vi "Test 100000 Log Writes.vi"(11 "Test Case In":refnum<class "File Sink.lvclass">) -> (0 "error out":errorcluster, 3 "Test Case Out":refnum<class "File Sink.lvclass">)   [LabVIEW 2020, in "Testing.lvlib" / "File Sink.lvclass"]
uses:
  File Sink.lvclass
  C:/Program Files (x86)/National Instruments/LabVIEW 2020/vi.lib/Astemes/LUnit/Test Case.lvclass
  Source/Type Defs/Debug Level.ctl
  <vilib>/Astemes/LUnit/Test Case.lvclass/Test Case.ctl
  0e3525c7-7213-410e-b7d5-902f6b8fb3e7.vi
  7c7b706d-9091-48de-aeff-4f50f38094d5.vi
  <vilib>/Astemes/LUnit/Core/LUnit Test Case/Private/Append Pass Result.vi
  <vilib>/Astemes/LUnit/Core/LUnit Test Case/Private/Append Fail Result.vi
  0e3525c7-7213-410e-b7d5-902f6b8fb3e7.vi/9c5d11cd-9439-4240-a1ee-d9baace9c924.vi
  7c7b706d-9091-48de-aeff-4f50f38094d5.vi/9c5d11cd-9439-4240-a1ee-d9baace9c924.vi
  <vilib>/Astemes/LUnit/Core/LUnit Test Case/Private/Run In UI.vi
  <vilib>/Utility/error.llb/Clear Errors.vi
  Source/Sinks/File Sink/File Sink.lvclass
  C:/Users/hughe_cx/Documents/05_repos/LVLog/Source/Sinks/Sink/Sink.lvclass
  Source/LV Log.lvlib
  Source/Logger/Logger.lvclass
  Testing.lvlib
  <vilib>/Astemes/LUnit/Test Case.lvclass
panel:
  out "Iteration (of 100000)":i32
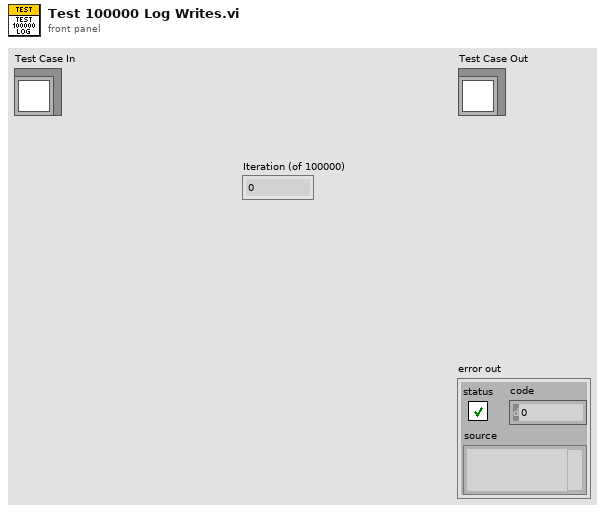
[diagram p1: front panel]
types:
  T1 = typedef "LV Log.lvlib/Debug Level.ctl" = enum16{"DEFAULT", "DEBUG", "INFO", "WARN", "ERROR", "FATAL"}
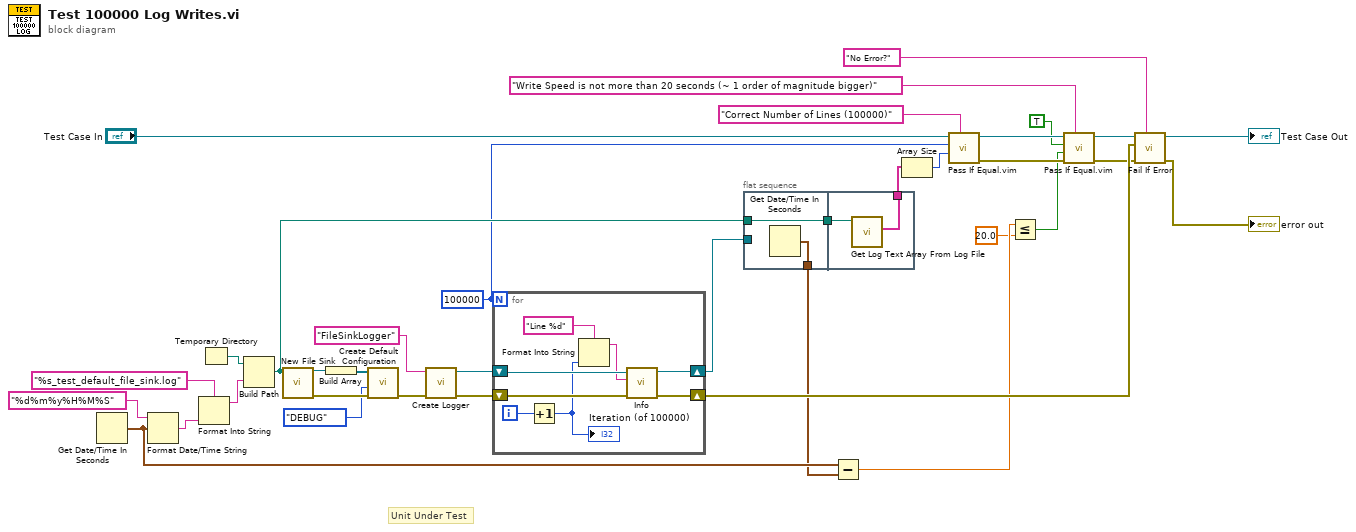
[diagram p0: block diagram]
diagram:
  w13 = 100000
  # "Unit Under Test"
  n1 = Get Date/Time In Seconds() -> (seconds since 1Jan1904=w7:timestamp)
  n2 = Format Date/Time String(time format string (%c)="%d%m%y%H%M%S", seconds (now)=w7) -> (date/time string=w28:string)  [unwired: 1 in]
  n3 = Format Into String(format string="%s_test_default_file_sink.log", w28) -> (resulting string=w30:string)  [unwired: 2 in, 1 out]
  n4 = Temporary Directory() -> (w32:path)
  n5 = Build Path(base path=w32, name or relative path=w30) -> (appended path=w23:path)
  n6 = call "New File Sink.vi"("File Path"=w23) -> ("error out"=w35:errorcluster, "File Sink out"=w33:refnum<class "File Sink.lvclass">)  [unwired: 9 in]
  n7 = Build Array(w33) -> (w34:refnum<class "File Sink.lvclass">[])
  n8 = call "Create Default Configuration.vi"("Sinks"=w34, "Debug Level in"=Debug_Level."DEBUG", "error in (no error)"=w35) -> ("error out"=w36:errorcluster)  [unwired: 7 in]
  n9 = call "Create Logger.vi"("error in (no error)"=w36, "Name"="FileSinkLogger") -> ("error out"=w26:errorcluster, "Logger out"=w25:refnum<class "Logger.lvclass">)  [unwired: 8 in]
  n10 = for {
    N: w13 -> [_]
    shift-right: [w41] -> w22
    shift-left: w25 -> [w43]
    shift-right: [w42] -> w18
    shift-left: w26 -> [w44]
    i -> [w38]
    n11 = Increment(x=w38) -> (x+1=w37:i32)
    "Iteration (of 100000)" <- w37
    n12 = Format Into String(format string="Line %d" ("Log Text"), w37) -> (resulting string=w39:string)  [unwired: 2 in, 1 out]
    n13 = call "Info.vi"("error in (no error)"=w44, "Log Text"=w39, "Logger in"=w43) -> ("error out"=w42:errorcluster, "Logger out"=w41:refnum<class "Logger.lvclass">)  [unwired: 6 in, 1 out]
  }
  n14 = flat-sequence {
    tunnel: w22 -> [_]
    tunnel: w23 -> [w46]
    tunnel: [w46] -> w8
    tunnel: [w45] -> w6
    tunnel: [w48] -> w21
    tunnel: w8 -> [w47]
    frame #0 {
      n15 = Get Date/Time In Seconds() -> (seconds since 1Jan1904=w45:timestamp)
    }
    frame #1 {
      n16 = call "Get Log Text Array From Log File.vi"("Log File Path in"=w47) -> ("Log Text Array"=w48:string[])  [unwired: 8 in, 2 out]
    }
  }
  n17 = Subtract(x=w7, y=w6) -> (x-y=w4:dbl)
  n18 = Array Size(array=w21) -> (size(s)=w20:i32)
  n19 = call "Pass If Equal.vim"("Description"="Correct Number of Lines (100000)", "Actual"=w20, "Expected"=w13, "LUnit Test Case In"="Test Case In") -> ("error out"=w10:errorcluster, "LUnit Test Case Out"=w12:refnum<class "File Sink.lvclass">)  [unwired: 6 in]
  n20 = Less Or Equal?(x=w4, y=20.0) -> (x <= y?=w2:bool)
  n21 = call "Pass If Equal.vim"("Description"="Write Speed is not more than 20 seconds (~ 1 order of magnitude bigger)", "error in (no error)"=w10, "Actual"=w2, "Expected"=TRUE, "LUnit Test Case In"=w12) -> ("error out"=w9:errorcluster, "LUnit Test Case Out"=w11:refnum<class "File Sink.lvclass">)  [unwired: 5 in]
  n22 = call <vilib>:"Fail If Error.vi"("Description"="No Error?", "error in (no error)"=w9, "Assert error"=w18, "LUnit Test Case In"=w11) -> ("error out"=→"error out":errorcluster, "LUnit Test Case Out"=→"Test Case Out":refnum<class "File Sink.lvclass">)  [unwired: 6 in]
